vi "Load Monitor Data.vi"(0 "SPU":refnum<k24>, 5 "PowerMonitorType":enum16{"DAQ", "MPM_220", "TSL_LOGG"}(ring), 7 "TSL":refnum<k24>, 9 "MPM":refnum<k24>[](array[refnum]), 11 "error in (no error)":errorcluster) -> (4 "trigger":sgl[](array[numeric]), 6 "monitor":sgl[](array[numeric]), 15 "error out":errorcluster)   [LabVIEW 2017]
uses:
  D:/test/ILSTS/LV_IL/LV_IL_Sample_x86/DLL/InstrumentDLL.dll
  DLL/InstrumentDLL.dll
  Share/Sweep_Speed.vi
  Share/Acctual_Step.vi
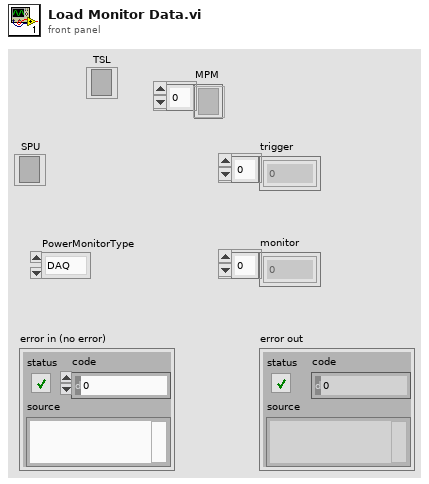
[diagram p1: front panel]
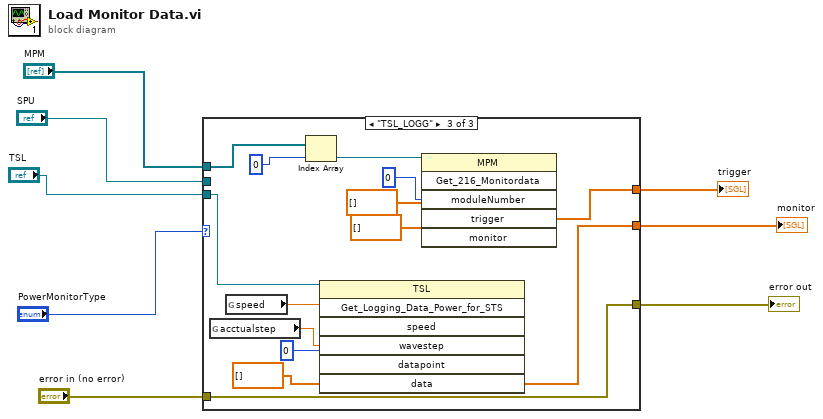
[diagram p0: block diagram]
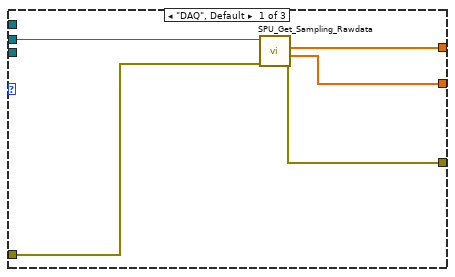
[diagram p2: hidden frame]
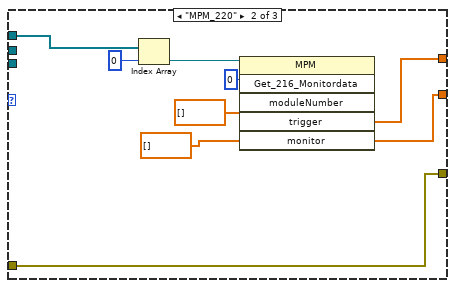
[diagram p3: hidden frame]
diagram:
  n1 = case shown="\"TSL_LOGG\"" "PowerMonitorType" {
    tunnel: "error in (no error)" -> [w13 w15 w23]
    tunnel: "SPU" -> [w12 _ _]
    tunnel: [w11 w15 w23] -> w6
    tunnel: [w10 w17 w30] -> w5
    tunnel: [w9 w16 w26] -> w4
    tunnel: "MPM" -> [_ w22 w31]
    tunnel: "TSL" -> [_ _ w29]
    frame "DAQ", Default {
      n2 = call "SPU_Get_Sampling_Rawdata.vi"("错误输入（无错误）"=w13, "SPU"=w12) -> ("error out"=w11:errorcluster, "monitor"=w9:sgl[], "trigger"=w10:sgl[])  [unwired: 5 in, 1 out]
    }
    frame "MPM_220" {
      n3 = Index Array(array=w22, index=0) -> (element=w20:refnum<k24>)
      n4 = invoke class="MPM" method="Get_216_Monitordata"(reference=w20, "moduleNumber"=0, "trigger"=sgl[] [], "monitor"=sgl[] []) -> ("trigger"=w17:sgl[], "monitor"=w16:sgl[])  [unwired: 2 in, 4 out]
    }
    frame "TSL_LOGG" {
      n5 = global read "Acctual_Step.vi" "acctualstep"() -> (w27:dbl)
      n6 = global read "Sweep_Speed.vi" "speed"() -> (w28:dbl)
      n7 = Index Array(array=w31, index=0) -> (element=w36:refnum<k24>)
      n8 = invoke class="TSL" method="Get_Logging_Data_Power_for_STS"(reference=w29, "speed"=w28, "wavestep"=w27, "datapoint"=0, "data"=sgl[] []) -> ("data"=w26:sgl[])  [unwired: 2 in, 6 out]
      n9 = invoke class="MPM" method="Get_216_Monitordata"(reference=w36, "moduleNumber"=0, "trigger"=sgl[] [], "monitor"=sgl[] []) -> ("trigger"=w30:sgl[])  [unwired: 2 in, 5 out]
    }
  }
  "error out" <- w6
  "trigger" <- w5
  "monitor" <- w4
